vi "Tabelle erstellen.vi"() -> (3 "Tabelle":T2[][](array[typedef]))   [LabVIEW 2020, in "EPA 1065.lvlib" / "Interference verificaton 1065-366.lvlib"]
uses:
  Interference verificaton 1065-366.lvlib
  Visualisierungs Elemente/String - Ausgabefeld.ctl
  Modus.ctl
  Aktion FGV Interference.ctl
  Seiten/FT-IR/FGV FT-IR Gasliste Aktionen.ctl
  Aktion Index uebersetzten.ctl
  Sprachverwaltung/FGV Aktion Tabelle zerlegen.ctl
  Seiten/FT-IR/FT-IR.lvlib
  Allgemein/allgemeine Sub-VIs.lvlib
  Sprachverwaltung/Sprachverwaltung.lvlib
panel:
  in  "Modus 2":T1 caption="Modus:" items=["Messen", "CG zu Entnahmestelle"]
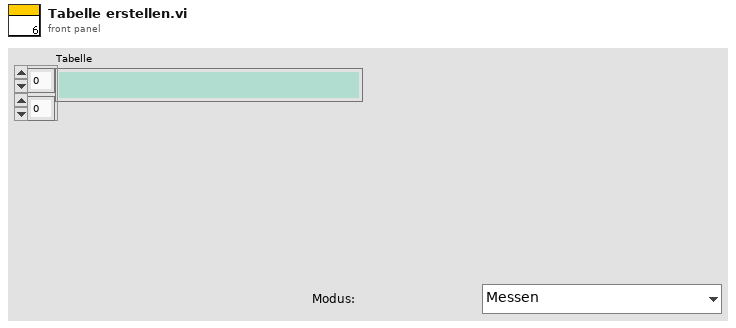
[diagram p1: front panel]
types:
  T1 = typedef "EPA 1065.lvlib/Interference verificaton 1065-366.lvlib/Modus.ctl" = u16
  T2 = typedef "String - Ausgabefeld.ctl" = string
  T3 = typedef "Sprachverwaltung.lvlib/FGV Aktion Tabelle zerlegen.ctl" = enum16{"laden", "vereinzeln", "speichern"}
  T4 = typedef "EPA 1065.lvlib/Interference verificaton 1065-366.lvlib/Aktion Index uebersetzten.ctl" = enum16{"lesen", "schreiben", "auswerten"}
  T5 = typedef "FT-IR.lvlib/FGV FT-IR Gasliste Aktionen.ctl" = enum16{"lesen", "Gasliste FT-IR", "Gasliste ausgelesen", "laden", "speichern", "löschen"}
  T6 = typedef "EPA 1065.lvlib/Interference verificaton 1065-366.lvlib/Aktion FGV Interference.ctl" = enum16{"Lesen", "TestKonfig", "TestSetting", "Einheiten", "Ergebnis", "Laden", "Tabelle", "Speichern", "löschen"}
  T7 = typedef "EPA 1065.lvlib/Interference verificaton 1065-366.lvlib/TestKonfig.ctl" = cluster{"CH4:":u16, "Ethane:":u16, "NMHC:":u16, "NMNEHC:":u16, "Komp 1 aktiv:":bool, "Komp 2 aktiv:":bool, "Komp 3 aktiv:":bool, "Komp 4 aktiv:":bool, "Modus":T1, "CG Aufschaltzeit:":dbl, "Interferent 1: CO2":u16, "Interferent 2: H2O":u16, "Interferent 3: CH4":u16, "Interferent 4: C2H6 / C3H8":u16, "Gasflaschen Nr.:":string, "Gasflaschen Nr.: 3":string, "Gasflaschen Nr.: 4":string, "Inter 1 aktiv":bool, "Inter 2 aktiv":bool, "Inter 3 aktiv":bool, "Inter 4 aktiv":bool, "Accuracy":string, "Accuracy 3":string, "Accuracy 4":string, "Konzentration 1:":dbl, "Konzentration 2:":dbl, "Konzentration 3:":dbl, "Konzentration 4:":dbl, "Flow weighted mean 1:":dbl, "Flow weighted mean 2:":dbl, "Flow weighted mean 3:":dbl, "Flow weighted mean 4:":dbl}
  T8 = typedef "EPA 1065.lvlib/Interference verificaton 1065-366.lvlib/Ergebnis.ctl" = cluster{"Interferent 1":sgl, "Interferent 2":sgl, "Interferent 3":sgl, "Interferent 4":sgl, "Komponente 1":sgl, "Komponente 2":sgl, "Komponente 3":sgl, "Komponente 4":sgl}
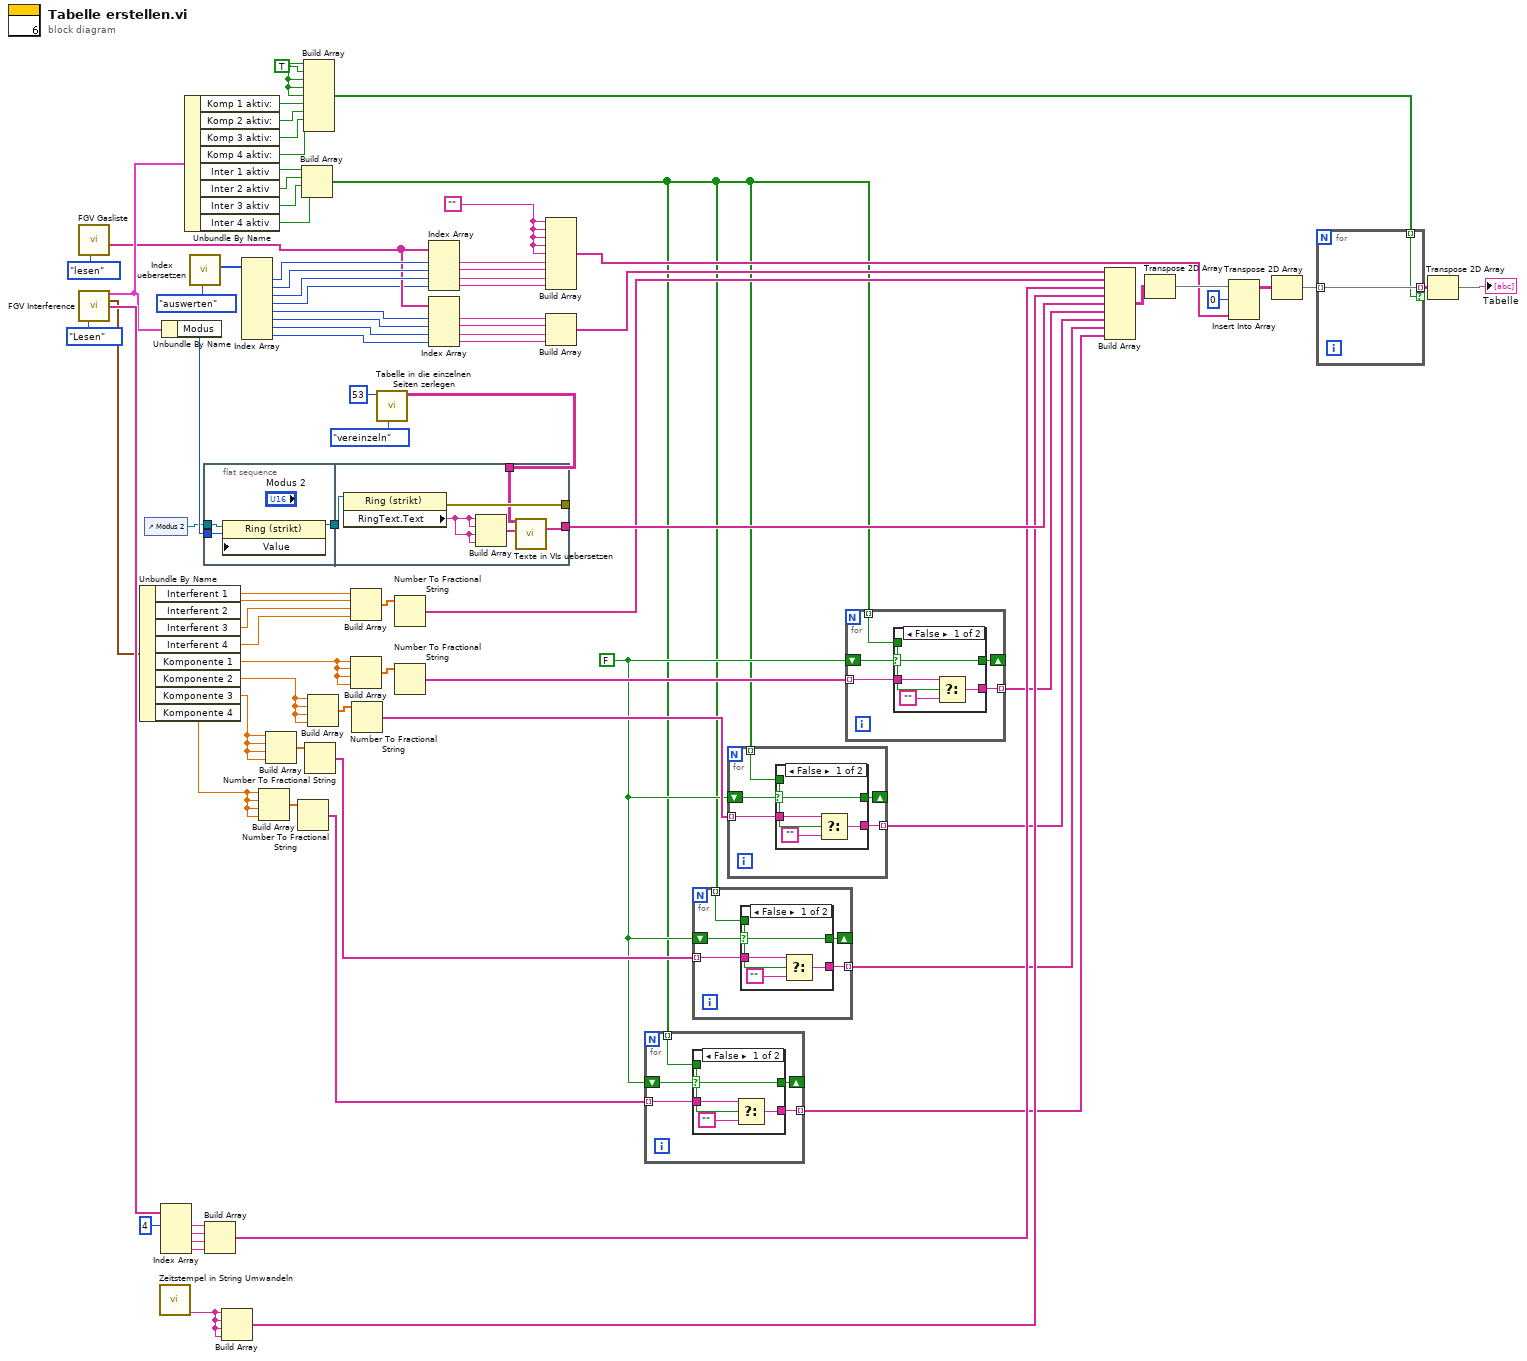
[diagram p0: block diagram]
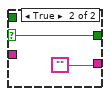
[diagram p2: hidden frame]
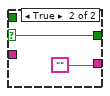
[diagram p3: hidden frame]
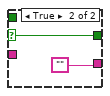
[diagram p4: hidden frame]
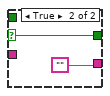
[diagram p5: hidden frame]
diagram:
  w20 = TRUE
  w32 = ""
  w12 = FALSE
  n1 = call "FGV Gasliste.vi"("Aktionen"=FGV_FT-IR_Gasliste_Aktionen."lesen") -> ("Aktuelle Gasliste gesamt"=w37:T2[])  [unwired: 8 in, 2 out]
  n2 = call "FGV Interference.vi"("Aktion FGV Interference"=Aktion_FGV_Interference."Lesen") -> ("TestKonfig"=w60:T7, "Ergebnis"=w69:T8, "Êinheiten"=w70:string[])  [unwired: 9 in, 3 out]
  n3 = Unbundle By Name(w69) -> ("Interferent 1"=w74:sgl, "Interferent 2"=w75:sgl, "Interferent 3"=w76:sgl, "Interferent 4"=w64:sgl, "Komponente 1"=w52:sgl, "Komponente 2"=w50:sgl, "Komponente 3"=w47:sgl, "Komponente 4"=w9:sgl)
  n4 = control-ref of="Modus 2"() -> (w55:refnum<vi>)
  n5 = call "Zeitstempel in String Umwandeln.vi"() -> ("Zeitstempel"=w63:string)  [unwired: 10 in, 1 out]
  n6 = Index Array(array=w70, index #1=4 ("Index")) -> (element #1=w29:string, element #2=w28:string, element #3=w27:string, element #4=w26:string)  [unwired: 3 in]
  n7 = Unbundle By Name(w60) -> ("Modus"=w81:T1)
  n8 = Unbundle By Name(w60) -> ("Komp 1 aktiv:"=w23:bool, "Komp 2 aktiv:"=w22:bool, "Komp 3 aktiv:"=w21:bool, "Komp 4 aktiv:"=w13:bool, "Inter 1 aktiv"=w59:bool, "Inter 2 aktiv"=w58:bool, "Inter 3 aktiv"=w57:bool, "Inter 4 aktiv"=w56:bool)
  n9 = call "Index uebersetzen.vi"("Aktion"=Aktion_Index_uebersetzten."auswerten") -> ("Komponenten"=w53:i32[])  [unwired: 9 in, 1 out]
  n10 = flat-sequence {
    tunnel: w81 -> [w86]
    tunnel: [w85] -> w66
    tunnel: w55 -> [w84]
    tunnel: [w92] -> _
    tunnel: [w88] -> w82
    tunnel: w66 -> [w91]
    tunnel: w14 -> [w87]
    frame #0 {
      n11 = property class="Ring (strikt)"(reference=w84, "Value"=w86) -> (reference out=w85:refnum<vi>)  [unwired: 1 in, 1 out]
    }
    frame #1 {
      n12 = property on="Eigenschaftsknoten" class="Ring (strikt)"(reference=w91) -> (error out=w92:errorcluster, "RingText.Text"=w90:string)  [unwired: 1 in, 1 out]
      n13 = Build Array(w90, w90, w90, w90) -> (w89:string[])
      n14 = call "Texte in VIs uebersetzen.vi"("Sprachliste"=w87, "String-Array zum Übersetzen"=w89) -> ("String-Array zum Übersetzen"=w88:string[])  [unwired: 9 in, 4 out]
    }
  }
  n15 = Build Array(w29, w28, w27, w26) -> (w79:string[])
  n16 = Build Array(w63, w63, w63, w63) -> (w80:string[])
  n17 = Index Array(array=w53) -> (element #1=w43:i32, element #2=w42:i32, element #3=w41:i32, element #4=w6:i32, element #5=w4:i32, element #6=w3:i32, element #7=w2:i32, element #8=w1:i32)  [unwired: 8 in]
  n18 = Build Array(w9, w9, w9, w9) -> (w10:sgl[])
  n19 = Build Array(w47, w47, w47, w47) -> (w46:sgl[])
  n20 = Number To Fractional String(number=w10) -> (F-format string=w8:string[])  [unwired: 3 in]
  n21 = Build Array(w59, w58, w57, w56) -> (w11:bool[])
  n22 = Build Array(w20, w20, w20, w20, w20, w23, w22, w21, w13) -> (w19:bool[])
  n23 = Number To Fractional String(number=w46) -> (F-format string=w45:string[])  [unwired: 3 in]
  n24 = Build Array(w50, w50, w50, w50) -> (w51:sgl[])
  n25 = Build Array(w74, w75, w76, w64) -> (w77:sgl[])
  n26 = Build Array(w52, w52, w52, w52) -> (w65:sgl[])
  n27 = Number To Fractional String(number=w51) -> (F-format string=w49:string[])  [unwired: 3 in]
  n28 = call "Tabelle in die einzelnen Seiten zerlegen.vi"("Aktion"=FGV_Aktion_Tabelle_zerlegen."vereinzeln", "Index (Seite)"=53) -> ("Sprachliste"=w14:string[][])  [unwired: 7 in, 2 out]
  n29 = Number To Fractional String(number=w77) -> (F-format string=w78:string[])  [unwired: 3 in]
  n30 = Number To Fractional String(number=w65) -> (F-format string=w62:string[])  [unwired: 3 in]
  n31 = Index Array(array=w37, index #1=w43, index #2=w42, index #3=w41, index #4=w6) -> (element #1=w71:T2, element #2=w72:T2, element #3=w73:T2, element #4=w5:T2)
  n32 = Index Array(array=w37, index #1=w4, index #2=w3, index #3=w2, index #4=w1) -> (element #1=w40:T2, element #2=w39:T2, element #3=w38:T2, element #4=w31:T2)
  n33 = Build Array(w32, w32, w32, w32, w32, w71, w72, w73, w5) -> (w34:T2[])
  n34 = Build Array(w40, w39, w38, w31) -> (w36:T2[])
  n35 = for {
    tunnel: w8 -> [w96] mode=indexing
    tunnel: [w97] -> w7 mode=indexing
    tunnel: w11 -> [w95] mode=indexing
    shift-right: [w93] -> _
    shift-left: w12 -> [w94]
    n36 = case shown="False" w94 {
      selector: w94 -> [_ w103]
      tunnel: [w101 ""] -> w97
      tunnel: w96 -> [w100 _]
      tunnel: w95 -> [w98 _]
      tunnel: [w98 w103] -> w93
      frame False {
        n37 = Select(t=w100, s=w98, f="") -> (s? t:f=w101:string)
      }
      frame True {
      }
    }
  }
  n38 = for {
    tunnel: w45 -> [w107] mode=indexing
    tunnel: [w108] -> w44 mode=indexing
    tunnel: w11 -> [w106] mode=indexing
    shift-right: [w104] -> _
    shift-left: w12 -> [w105]
    n39 = case shown="False" w105 {
      selector: w105 -> [_ w114]
      tunnel: [w112 ""] -> w108
      tunnel: w107 -> [w111 _]
      tunnel: w106 -> [w109 _]
      tunnel: [w109 w114] -> w104
      frame False {
        n40 = Select(t=w111, s=w109, f="") -> (s? t:f=w112:string)
      }
      frame True {
      }
    }
  }
  n41 = for {
    tunnel: w49 -> [w118] mode=indexing
    tunnel: [w119] -> w48 mode=indexing
    tunnel: w11 -> [w117] mode=indexing
    shift-right: [w115] -> _
    shift-left: w12 -> [w116]
    n42 = case shown="False" w116 {
      selector: w116 -> [_ w125]
      tunnel: [w123 ""] -> w119
      tunnel: w118 -> [w122 _]
      tunnel: w117 -> [w120 _]
      tunnel: [w120 w125] -> w115
      frame False {
        n43 = Select(t=w122, s=w120, f="") -> (s? t:f=w123:string)
      }
      frame True {
      }
    }
  }
  n44 = for {
    tunnel: w62 -> [w129] mode=indexing
    tunnel: [w130] -> w61 mode=indexing
    tunnel: w11 -> [w128] mode=indexing
    shift-right: [w126] -> _
    shift-left: w12 -> [w127]
    n45 = case shown="False" w127 {
      selector: w127 -> [_ w136]
      tunnel: [w134 ""] -> w130
      tunnel: w129 -> [w133 _]
      tunnel: w128 -> [w131 _]
      tunnel: [w131 w136] -> w126
      frame False {
        n46 = Select(t=w133, s=w131, f="") -> (s? t:f=w134:string)
      }
      frame True {
      }
    }
  }
  n47 = Build Array(w36, w78, w79, w80, w82, w61, w48, w44, w7) -> (w83:T2[][])
  n48 = Transpose 2D Array(2D array=w83) -> (transposed array=w35:T2[][])
  n49 = Insert Into Array(array=w35, index (row)=0 ("Index (Zeile)"), new element=w34) -> (w24:T2[][])  [unwired: 1 in]
  n50 = Transpose 2D Array(2D array=w24) -> (transposed array=w18:T2[][])
  n51 = for {
    tunnel: [w138] -> w25 mode=indexing if=w137
    tunnel: w18 -> [w138] mode=indexing
    tunnel: w19 -> [w137] mode=indexing
  }
  n52 = Transpose 2D Array(2D array=w25) -> (transposed array=→"Tabelle":T2[][])
